vi "DW-82 Control.vi"(8 "error in (no error)":errorcluster caption="错误输入（无错误）", 9 "Test Type":enum16{"Voltage", "Current", "Power", "Frq"}(ring), 10 "Address":u8=3, 11 "MyIndex":u8) -> (0 "error IO":errorcluster, 3 "Measure Value":dbl)   [LabVIEW 2015]
panel:
  out "VISA":refnum<visa-resource-name> caption="VISA资源名称输出"
  out "OK?":bool
  out "StrOut":string
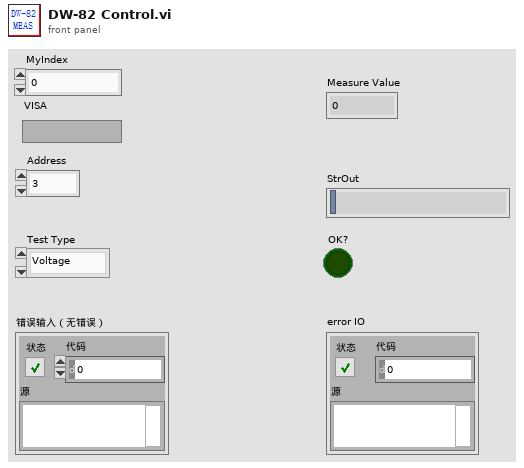
[diagram p1: front panel]
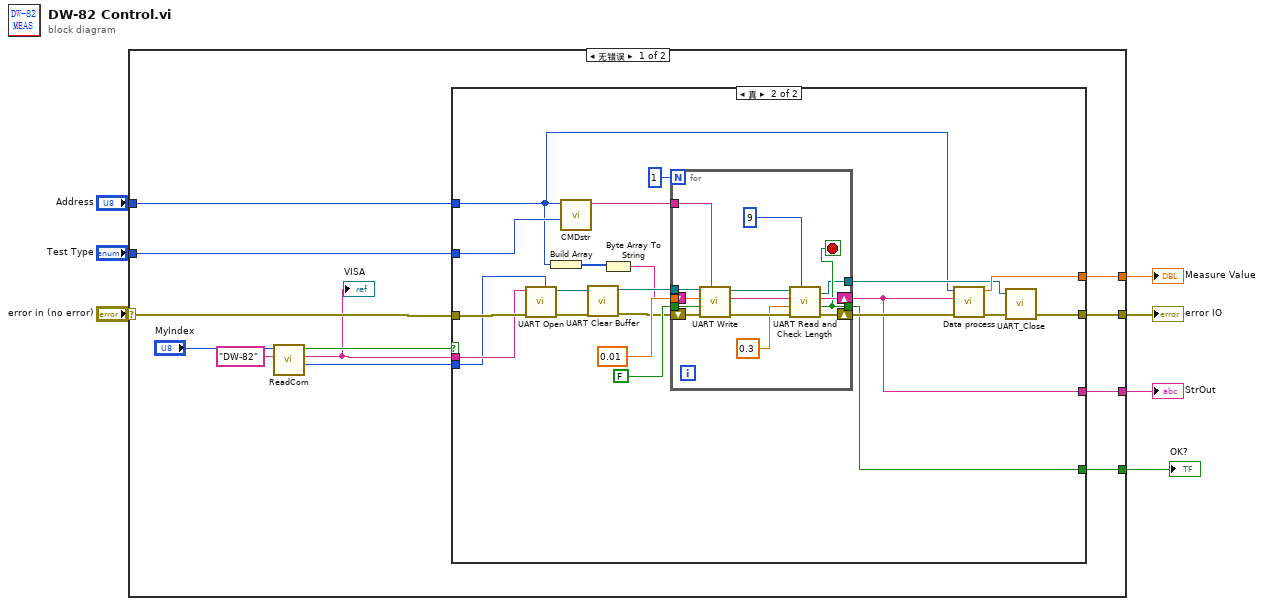
[diagram p0: block diagram]
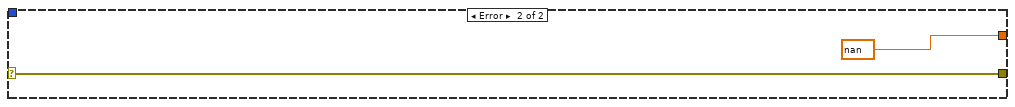
[diagram p3: hidden frame]
diagram:
  n1 = case shown="无错误" "error in (no error)" {
    selector: "error in (no error)" -> [w16 w57]
    tunnel: "Address" -> [w18 _]
    tunnel: [w17 nan ("Data_Float")] -> w4
    tunnel: [w15 w57] -> w5
    tunnel: [w19 _] -> w3
    tunnel: "Test Type" -> [w14 _]
    tunnel: [w11 _] -> w1
    frame No Error {
      n2 = call "ReadCom.vi"("仪器名称"="DW-82", "MyIndex"="MyIndex") -> ("Baudrate"=w8:i32, "COM"=w9:string, "OK?"=w10:bool)  [unwired: 7 in]
      "VISA" <- w9
      n3 = case shown="真" w10 {
        tunnel: [_ w36] -> w19
        tunnel: w18 -> [_ w20]
        tunnel: [_ w31] -> w17
        tunnel: w16 -> [_ w29]
        tunnel: [_ w26] -> w15
        tunnel: w14 -> [_ w21]
        tunnel: [_ w24] -> w11
        tunnel: w9 -> [_ w23]
        tunnel: w8 -> [_ w22]
        frame False {
        }
        frame True {
          n4 = call "UART Open.vi"("baud rate (9600)"=w22, "error in"=w29, "VISA resource name"=w23) -> ("error out"=w28:errorcluster, "VISA resource name out"=w27:refnum<visa-resource-name>)  [unwired: 7 in]
          n5 = Build Array(w20) -> (w33:u8[])
          n6 = call "CMDstr.vi"("Test Type"=w21, "Address"=w20) -> ("CMD"=w38:string)  [unwired: 9 in]
          n7 = call "UART Clear Buffer.vi"("Error In"=w28, "VISA Resource In"=w27) -> ("Error Out"=w35:errorcluster, "VISA Resource Out"=w34:refnum<visa-resource-name>)  [unwired: 5 in]
          n8 = Byte Array To String(unsigned byte array=w33) -> (string=w32:string)
          n9 = for {
            N: 1 -> [_]
            tunnel: FALSE ("Add Return") -> [w55]
            tunnel: 0.01 ("Write Delay (s)") -> [w54]
            tunnel: w38 -> [w49]
            tunnel: w34 -> [w46]
            tunnel: [w43] -> w24
            shift-right: [w50] -> w39
            shift-left: w35 -> [w47]
            shift-right: [w48] -> w36
            shift-left: w32 -> [w44]
            tunnel: [w42] -> w25
            stop <- w43 stop-if-true
            n10 = call "UART Write.vi"("write buffer"=w49, "error in (no error)"=w47, "Add Return"=w55, "Write Delay (s)"=w54, "VISA Resource In"=w46) -> ("error out"=w53:errorcluster, "VISA Resource Out"=w52:refnum<visa-resource-name>)  [unwired: 2 in]
            n11 = call "UART Read and Check Length.vi"("Len"=u8 9, "error in (no error)"=w53, "TimeOut(s)"=0.3, "ExpectStr"=w44, "VISA Resource In"=w52) -> ("error out"=w50:errorcluster, "OK?"=w43:bool, "StrOut"=w48:string, "VISA Resource Out"=w42:refnum<visa-resource-name>)
          }
          n12 = call "Data process.vi"("error in"=w39, "Data Read"=w36, "Address"=w20) -> ("error IO"=w37:errorcluster, "V"=w31:dbl)  [unwired: 5 in, 2 out]
          n13 = call "UART_Close.vi"("error in (no error)"=w37, "VISA Resource In"=w25) -> ("error out"=w26:errorcluster)  [unwired: 3 in]
        }
      }
    }
    frame Error {
    }
  }
  "error IO" <- w5
  "Measure Value" <- w4
  "StrOut" <- w3
  "OK?" <- w1
